vi "Get_Displacement.vi"(5 "Device Number":T1, 7 "Update":bool) -> (2 "Displacement":T2)   [LabVIEW 2016]
doc: "This navX VI returns the velocity and displacement of the navX. This VI is only supported on firmware virsions newer than 2.2.xxx."
uses:
  TypeDefs/FRIC_navX_DecodeRegisterLengthClusterTypeDef_.ctl
  TypeDefs/Z900_navX_DeviceRegisters.ctl
  navX Library v2.lvlib
  TypeDefs/FRIC_navX_DeviceNumbersTypeDef.ctl
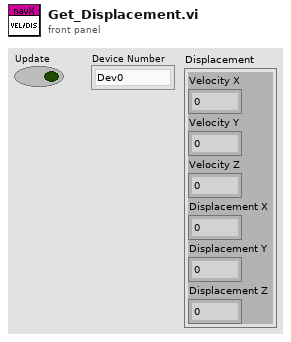
[diagram p1: front panel]
types:
  T1 = typedef "FRIC_navX_DeviceNumbersTypeDef.ctl" = enum16{"Dev0", "Dev1", "Dev2", "Dev3"}
  T2 = cluster{"Velocity X":dbl, "Velocity Y":dbl, "Velocity Z":dbl, "Displacement X":dbl, "Displacement Y":dbl, "Displacement Z":dbl}
  T3 = typedef "FRIC_navX_DecodeRegisterLengthClusterTypeDef_.ctl" = cluster{"Device Register":T4, "length":i32}[]
  T4 = typedef "navX Library v2.lvlib/Z900_navX_DeviceRegisters.ctl" = u8
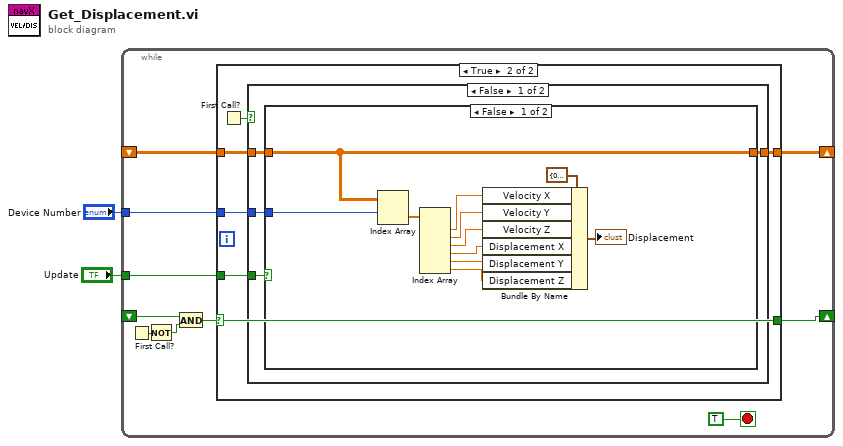
[diagram p0: block diagram]
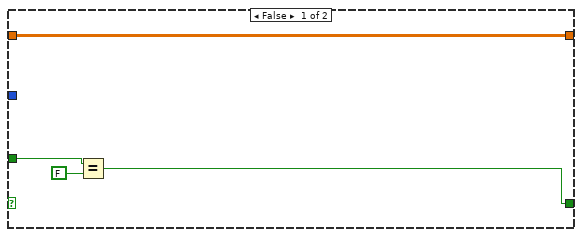
[diagram p2: hidden frame]
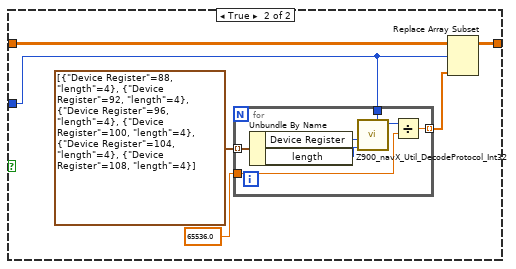
[diagram p3: hidden frame]
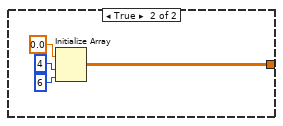
[diagram p4: hidden frame]
diagram:
  n1 = while {
    shift-right: [w12] -> _
    shift-left: _ -> [w10]
    tunnel: "Update" -> [w9]
    tunnel: "Device Number" -> [w8]
    shift-right: [w3] -> _
    shift-left: _ -> [w5]
    stop <- TRUE stop-if-true
    n2 = First Call?() -> (First Call?: T/F=w7:bool)
    n3 = Not(x=w7) -> (.not. x?=w6:bool)
    n4 = And(x=w5, y=w6) -> (x .and. y?=w4:bool)
    n5 = case shown="True" w4 {
      selector: w4 -> [_ w17]
      tunnel: [w13 w22] -> w12
      tunnel: w10 -> [w13 w21]
      tunnel: w9 -> [w15 w20]
      tunnel: w8 -> [_ w19]
      tunnel: [w14 w17] -> w3
      frame False {
        n6 = Equal?(x=w15, y=FALSE) -> (x = y?=w14:bool)
      }
      frame True {
        n7 = First Call?() -> (First Call?: T/F=w18:bool)
        n8 = case shown="False" w18 {
          tunnel: [w26 w51] -> w22
          tunnel: w21 -> [w25 _]
          tunnel: w20 -> [w23 _]
          tunnel: w19 -> [w24 _]
          frame False {
            n9 = case shown="False" w23 {
              tunnel: [w29 w38] -> w26
              tunnel: w25 -> [w29 w41]
              tunnel: w24 -> [w28 w39]
              frame False {
                n10 = Index Array(array=w29, index (row)=w28) -> (element=w31:dbl[])  [unwired: 1 in]
                n11 = Index Array(array=w31) -> (element #1=w32:dbl, element #2=w33:dbl, element #3=w34:dbl, element #4=w35:dbl, element #5=w36:dbl, element #6=w37:dbl)  [unwired: 6 in]
                n12 = Bundle By Name(cluster=T2 {"Velocity X"=0.0, "Velocity Y"=0.0, "Velocity Z"=0.0, "Displacement X"=0.0, "Displacement Y"=0.0, "Displacement Z"=0.0}, "Velocity X"=w32, "Velocity Y"=w33, "Velocity Z"=w34, "Displacement X"=w35, "Displacement Y"=w36, "Displacement Z"=w37) -> (→"Displacement":T2)
              }
              frame True {
                n13 = for {
                  tunnel: T3 [{"Device Register"=88, "length"=4}, {"Device Register"=92, "length"=4}, {"Device Register"=96, "length"=4}, {"Device Register"=100, "length"=4}, {"Device Register"=104, "length"=4}, {"Device Register"=108, "length"=4}] -> [w50] mode=indexing
                  tunnel: w39 -> [w47]
                  tunnel: 65536.0 ("y") -> [w45]
                  tunnel: [w44] -> w40 mode=indexing
                  n14 = Unbundle By Name(w50) -> ("Device Register"=w49:T4, "length"=w48:i32)
                  n15 = call "Z900_navX_Util_DecodeProtocol_Int32.vi"("Device Number"=w47, "length"=w48, "Device Register"=w49) -> ("Value"=w46:i32)  [unwired: 7 in]
                  n16 = Divide(x=w46, y=w45) -> (x/y=w44:dbl)
                }
                n17 = Replace Array Subset(array=w41, new element=w40, index (row)=w39) -> (w38:dbl[][])  [unwired: 1 in]
              }
            }
          }
          frame True {
            n18 = Initialize Array(0.0, 4 ("dimension size"), 6 ("dimension size")) -> (w51:dbl[][])
          }
        }
      }
    }
  }
